vi "Brushless DC IO.vi"(10 "Brushless DC Motor PWM":sgl min=-100 max=100, 11 "IO Cluster IN":T1) -> (0 "Error Out":errorcluster, 1 "BLDC Hall Effect Sensor State":u8, 2 "Brushless DC Motor Speed (RPM)":dbl, 3 "IO Cluster OUT":T1, 4 "Hall Effect Sensor Error":bool)   [LabVIEW 2019]
uses:
  Actuators IO Cluster.ctl
  <vilib>/Utility/error.llb/Error Cluster From Error Code.vi
  <vilib>/rvi/errors/niLvFpgaAdjustHostInterfaceError.vi
  <vilib>/rvi/interface/nirviReadWriteControl/nirviReadWriteControl.xnode
  NiFpgaLv.dll
  <vilib>/rvi/interface/Simulation/niFpgaSimulationCallBeginRW.vi
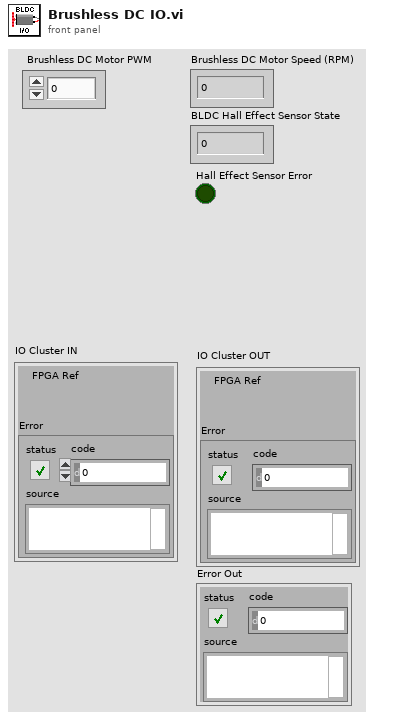
[diagram p1: front panel]
types:
  T1 = typedef "Actuators IO Cluster.ctl" = cluster{"Error":errorcluster, "FPGA Ref":refnum<k20>}
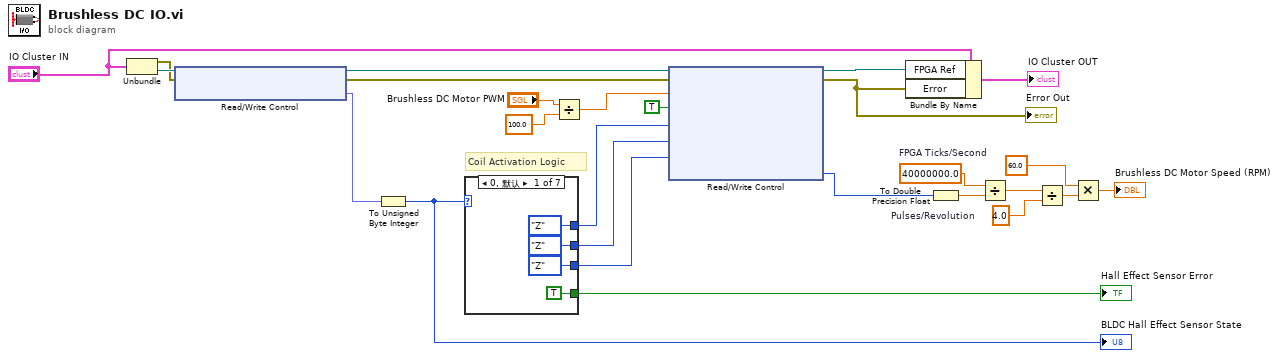
[diagram p0: block diagram]
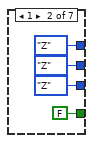
[diagram p2: hidden frame]
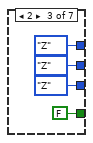
[diagram p3: hidden frame]
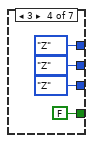
[diagram p4: hidden frame]
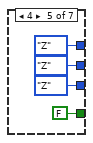
[diagram p5: hidden frame]
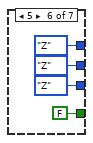
[diagram p6: hidden frame]
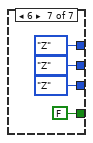
[diagram p7: hidden frame]
diagram:
  w22 = 4.0  # Pulses/Revolution
  w24 = 40000000.0  # FPGA Ticks/Second
  # "Coil Activation Logic"
  n1 = Unbundle("IO Cluster IN") -> ("Error"=w4:errorcluster, "FPGA Ref"=w5:refnum<k20>)
  n2 = xnode "Read/Write Control"("FPGA VI引用输入"=w5, "错误输入"=w4) -> ("FPGA VI引用输出"=w10:refnum<k20>, "错误输出"=w9:errorcluster, "BLDC Encoder RAW A/B/C"=w8:fxp<+,3,3>)
  n3 = To Unsigned Byte Integer(number=w8) -> (unsigned 8bit integer=w6:u8)
  "BLDC Hall Effect Sensor State" <- w6
  n4 = case shown="0, 默认" w6 {
    tunnel: [TRUE FALSE FALSE FALSE FALSE FALSE FALSE] -> w7
    tunnel: [enum16{"H", "L", "Z"}."Z" ("BLDC Drive Phase A") enum16{"H", "L", "Z"}."Z" ("BLDC Drive Phase A") enum16{"H", "L", "Z"}."Z" ("BLDC Drive Phase A") enum16{"H", "L", "Z"}."Z" ("BLDC Drive Phase A") enum16{"H", "L", "Z"}."Z" ("BLDC Drive Phase A") enum16{"H", "L", "Z"}."Z" ("BLDC Drive Phase A") enum16{"H", "L", "Z"}."Z" ("BLDC Drive Phase A")] -> w13
    tunnel: [enum16{"H", "L", "Z"}."Z" ("BLDC Drive Phase B") enum16{"H", "L", "Z"}."Z" ("BLDC Drive Phase B") enum16{"H", "L", "Z"}."Z" ("BLDC Drive Phase B") enum16{"H", "L", "Z"}."Z" ("BLDC Drive Phase B") enum16{"H", "L", "Z"}."Z" ("BLDC Drive Phase B") enum16{"H", "L", "Z"}."Z" ("BLDC Drive Phase B") enum16{"H", "L", "Z"}."Z" ("BLDC Drive Phase B")] -> w12
    tunnel: [enum16{"H", "L", "Z"}."Z" ("BLDC Drive Phase C") enum16{"H", "L", "Z"}."Z" ("BLDC Drive Phase C") enum16{"H", "L", "Z"}."Z" ("BLDC Drive Phase C") enum16{"H", "L", "Z"}."Z" ("BLDC Drive Phase C") enum16{"H", "L", "Z"}."Z" ("BLDC Drive Phase C") enum16{"H", "L", "Z"}."Z" ("BLDC Drive Phase C") enum16{"H", "L", "Z"}."Z" ("BLDC Drive Phase C")] -> w11
    frame 0, Default {
    }
    frame 1 {
    }
    frame 2 {
    }
    frame 3 {
    }
    frame 4 {
    }
    frame 5 {
    }
    frame 6 {
    }
  }
  "Hall Effect Sensor Error" <- w7
  n5 = Divide(x="Brushless DC Motor PWM", y=sgl 100.0) -> (x/y=w16:sgl)
  n6 = xnode "Read/Write Control"("FPGA VI引用输入"=w10, "错误输入"=w9, "BLDC PWM (0-1)"=w16, "LED BLDC"=TRUE ("LED DC Motor"), "BLDC Drive Phase A"=w13, "BLDC Drive Phase B"=w12, "BLDC Drive Phase C"=w11) -> ("FPGA VI引用输出"=w2:refnum<k20>, "错误输出"=w1:errorcluster, "BLDC Motor Tach Ticks"=w14:u32)
  "Error Out" <- w1
  n7 = Bundle By Name(cluster="IO Cluster IN", "FPGA Ref"=w2, "Error"=w1) -> (→"IO Cluster OUT":T1)
  n8 = To Double Precision Float(number=w14) -> (double precision float=w25:dbl)
  n9 = Divide(x=w24, y=w25) -> (x/y=w23:dbl)
  n10 = Divide(x=w23, y=w22) -> (x/y=w20:dbl)
  n11 = Multiply(x=60.0, y=w20) -> (x*y=→"Brushless DC Motor Speed (RPM)":dbl)
